vi "CO TCP Packet_v2.0.vi"(7 "TCP Packet Content":string, 13 "Data Array":string[](array[string])) -> (8 "TCP Binary Packet":string)   [LabVIEW 2014]
panel:
  out "array":string[](array[string])
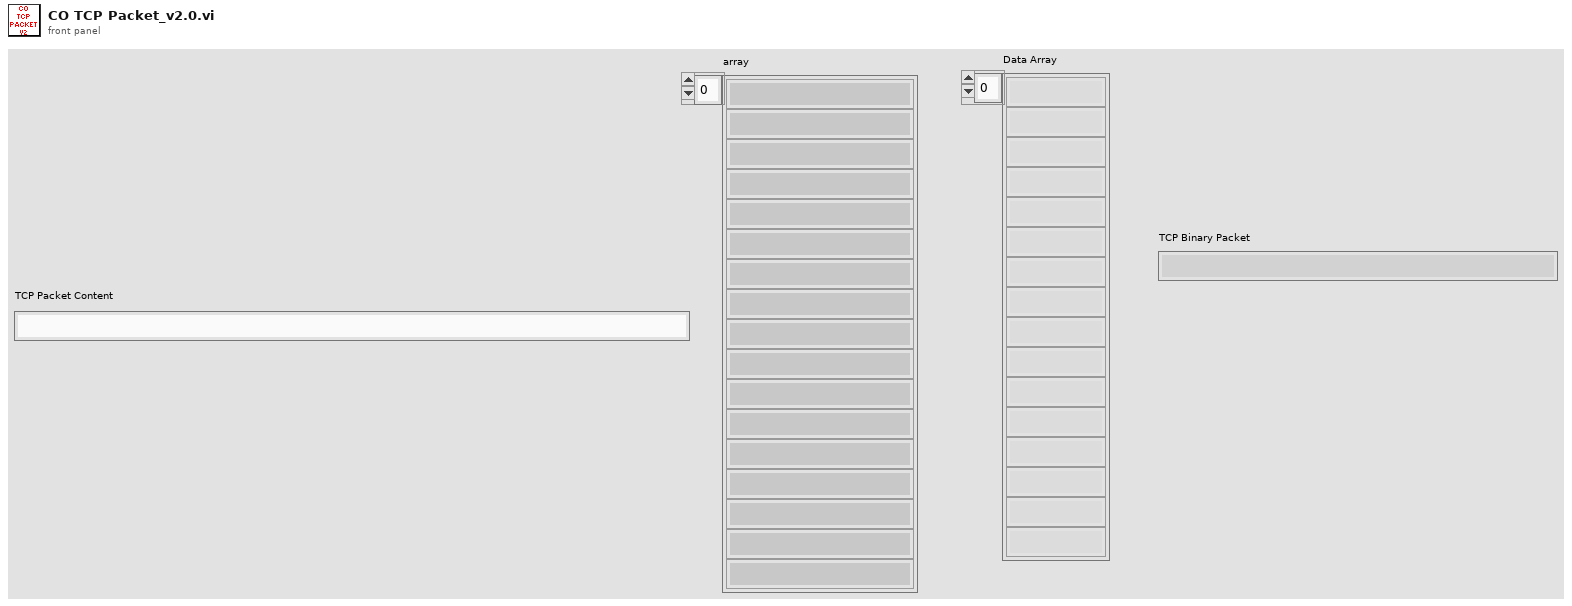
[diagram p1: front panel]
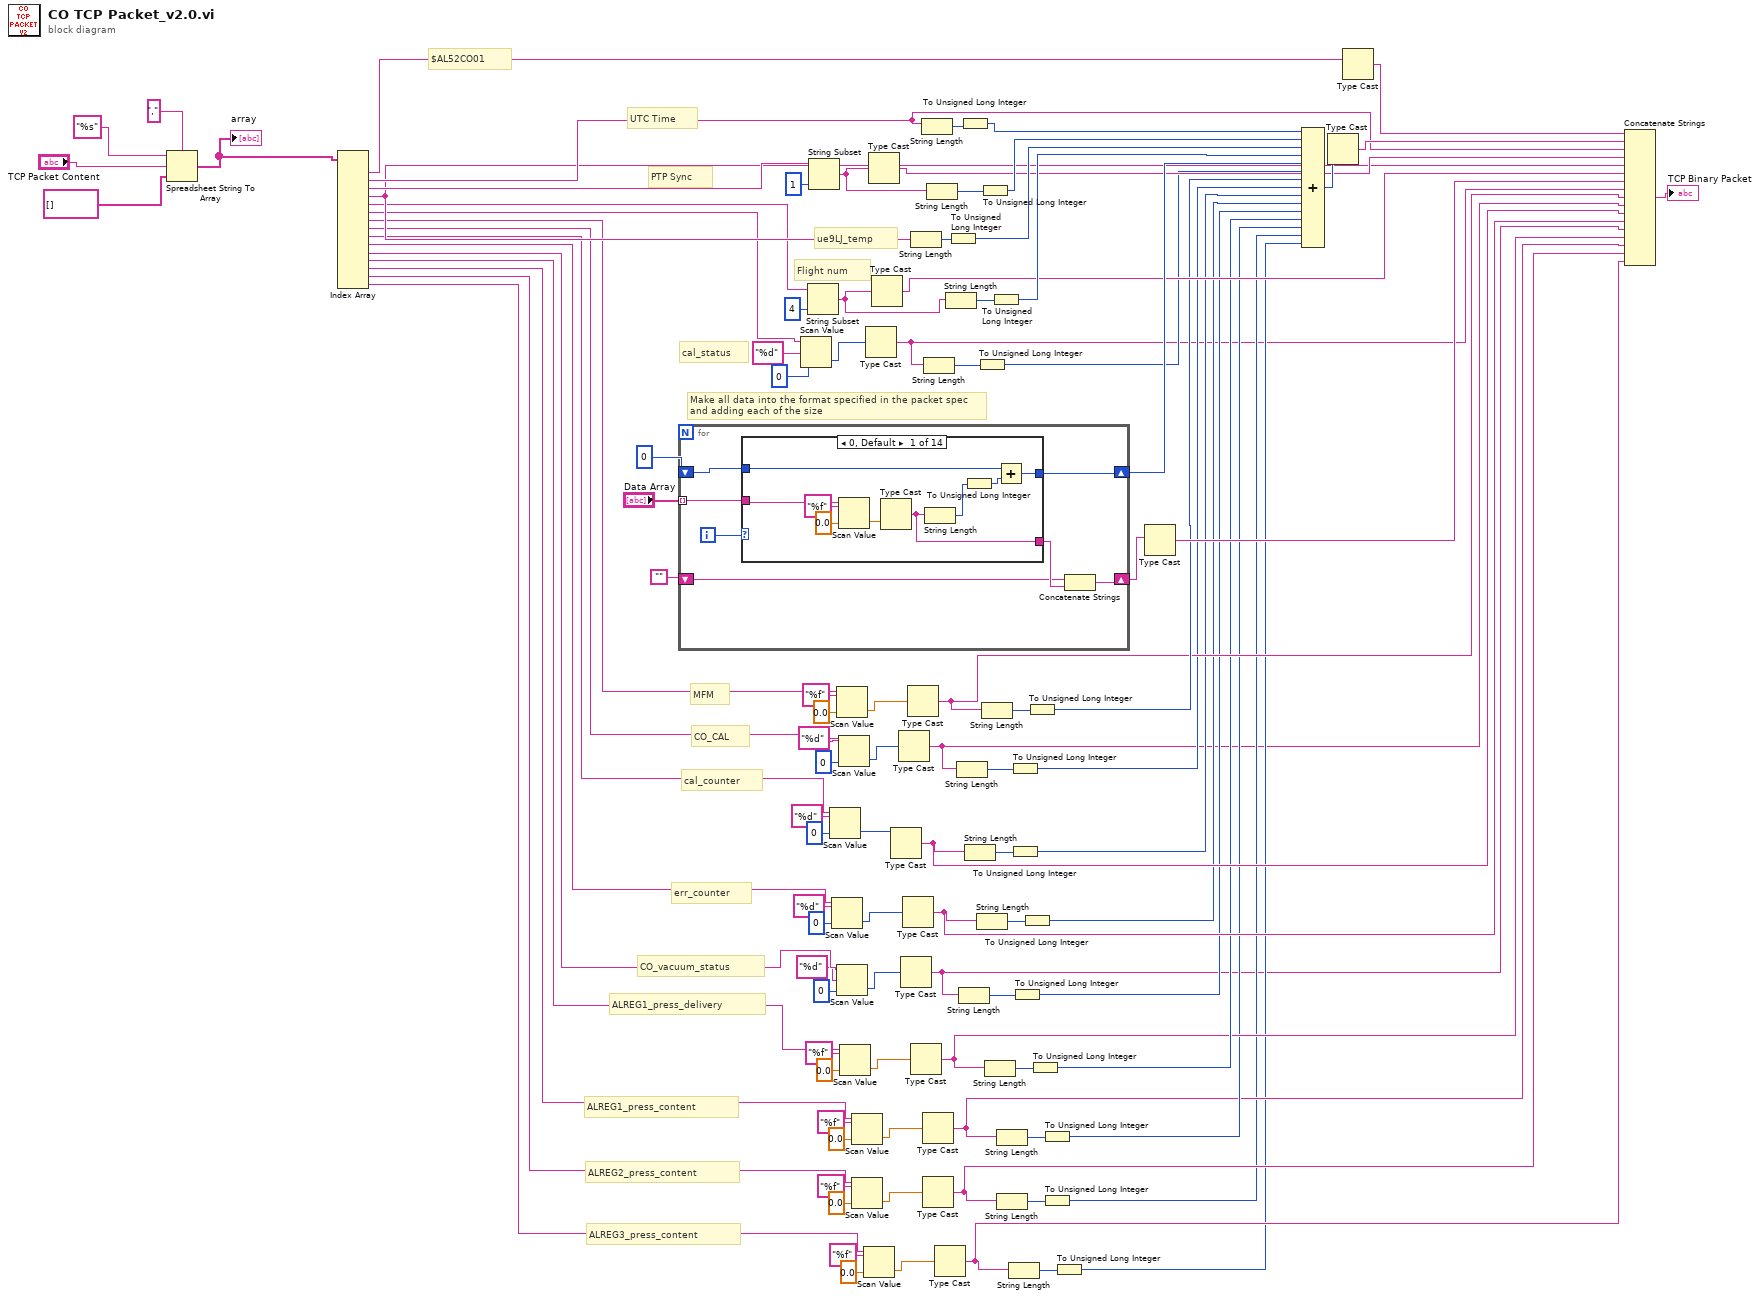
[diagram p0: block diagram]
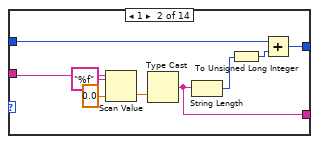
[diagram p2: hidden frame]
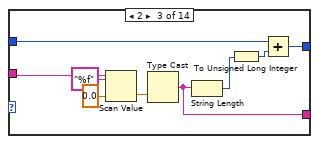
[diagram p3: hidden frame]
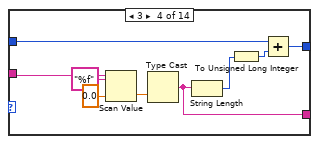
[diagram p4: hidden frame]
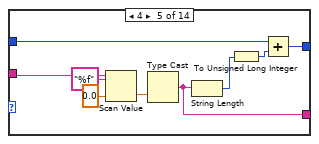
[diagram p5: hidden frame]
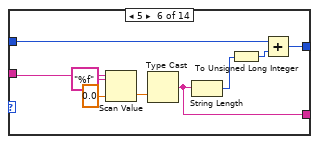
[diagram p6: hidden frame]
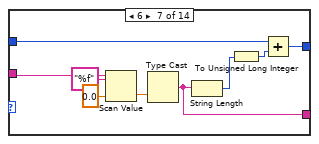
[diagram p7: hidden frame]
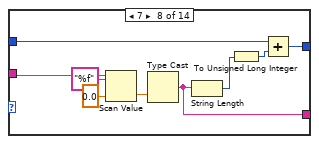
[diagram p8: hidden frame]
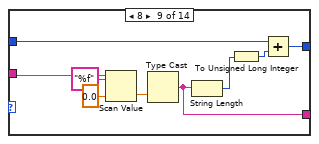
[diagram p9: hidden frame]
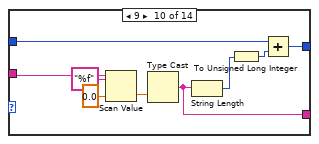
[diagram p10: hidden frame]
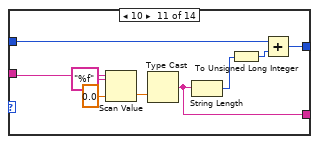
[diagram p11: hidden frame]
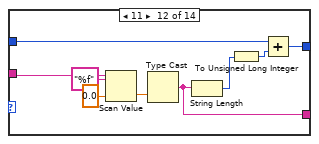
[diagram p12: hidden frame]
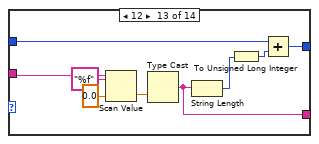
[diagram p13: hidden frame]
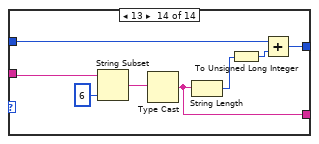
[diagram p14: hidden frame]
diagram:
  # "ALREG3_press_content"
  # "ALREG2_press_content"
  # "ALREG1_press_content"
  # "ALREG1_press_delivery"
  # "CO_vacuum_status"
  # "err_counter"
  # "cal_counter"
  # "CO_CAL"
  # "MFM"
  # "cal_status"
  # "Flight num"
  # "ue9LJ_temp"
  # "PTP Sync"
  # "UTC Time"
  # "$AL52CO01"
  # "Make all data into the format specified in the packet spec\nand adding each of the size"
  n1 = Spreadsheet String To Array(delimiter (Tab)=",", format string="%s", spreadsheet string="TCP Packet Content", array type (2D Dbl)=string[] []) -> (array=w74:string[])
  "array" <- w74
  n2 = Index Array(array=w74) -> (element #1=w73:string, element #2=w72:string, element #3=w71:string, element #4=w70:string, element #5=w69:string, element #6=w10:string, element #7=w64:string, element #8=w15:string, element #9=w34:string, element #10=w31:string, element #11=w4:string, element #12=w27:string, element #13=w24:string, element #14=w20:string, element #15=w18:string)  [unwired: 15 in]
  n3 = for {
    tunnel: "Data Array" -> [w110] mode=indexing
    shift-right: [w108] -> w92
    shift-left: u32 0 -> [w109]
    shift-right: [w107] -> w81
    shift-left: "" -> [w105]
    i -> [w111]
    n4 = case shown="0, Default" w111 {
      tunnel: w110 -> [w118 w127 w136 w145 w154 w163 w172 w181 w190 w199 w208 w217 w226 w230]
      tunnel: w109 -> [w116 w125 w134 w143 w152 w161 w170 w179 w188 w197 w206 w215 w224 w236]
      tunnel: [w113 w122 w131 w140 w149 w158 w167 w176 w185 w194 w203 w212 w221 w233] -> w108
      tunnel: [w112 w121 w130 w139 w148 w157 w166 w175 w184 w193 w202 w211 w220 w232] -> w106
      frame 0, Default {
        n5 = Scan Value(string=w118, format string="%f", default (0 dbl)=sgl 0.0 ("default (0 I32)")) -> (value=w120:sgl)  [unwired: 1 out]
        n6 = Type Cast(x=w120) -> (*(type *) &x=w112:string)  [unwired: 1 in]
        n7 = String Length(string=w112) -> (length=w115:i32)
        n8 = To Unsigned Long Integer(number=w115) -> (unsigned 32bit integer=w114:u32)
        n9 = Add(x=w116, y=w114) -> (x+y=w113:u32)
      }
      frame 1 {
        n10 = Scan Value(string=w127, format string="%f", default (0 dbl)=sgl 0.0 ("default (0 I32)")) -> (value=w129:sgl)  [unwired: 1 out]
        n11 = Type Cast(x=w129) -> (*(type *) &x=w121:string)  [unwired: 1 in]
        n12 = String Length(string=w121) -> (length=w124:i32)
        n13 = To Unsigned Long Integer(number=w124) -> (unsigned 32bit integer=w123:u32)
        n14 = Add(x=w125, y=w123) -> (x+y=w122:u32)
      }
      frame 2 {
        n15 = Scan Value(string=w136, format string="%f", default (0 dbl)=sgl 0.0 ("default (0 I32)")) -> (value=w138:sgl)  [unwired: 1 out]
        n16 = Type Cast(x=w138) -> (*(type *) &x=w130:string)  [unwired: 1 in]
        n17 = String Length(string=w130) -> (length=w133:i32)
        n18 = To Unsigned Long Integer(number=w133) -> (unsigned 32bit integer=w132:u32)
        n19 = Add(x=w134, y=w132) -> (x+y=w131:u32)
      }
      frame 3 {
        n20 = Scan Value(string=w145, format string="%f", default (0 dbl)=sgl 0.0 ("default (0 I32)")) -> (value=w147:sgl)  [unwired: 1 out]
        n21 = Type Cast(x=w147) -> (*(type *) &x=w139:string)  [unwired: 1 in]
        n22 = String Length(string=w139) -> (length=w142:i32)
        n23 = To Unsigned Long Integer(number=w142) -> (unsigned 32bit integer=w141:u32)
        n24 = Add(x=w143, y=w141) -> (x+y=w140:u32)
      }
      frame 4 {
        n25 = Scan Value(string=w154, format string="%f", default (0 dbl)=sgl 0.0 ("default (0 I32)")) -> (value=w156:sgl)  [unwired: 1 out]
        n26 = Type Cast(x=w156) -> (*(type *) &x=w148:string)  [unwired: 1 in]
        n27 = String Length(string=w148) -> (length=w151:i32)
        n28 = To Unsigned Long Integer(number=w151) -> (unsigned 32bit integer=w150:u32)
        n29 = Add(x=w152, y=w150) -> (x+y=w149:u32)
      }
      frame 5 {
        n30 = Scan Value(string=w163, format string="%f", default (0 dbl)=sgl 0.0 ("default (0 I32)")) -> (value=w165:sgl)  [unwired: 1 out]
        n31 = Type Cast(x=w165) -> (*(type *) &x=w157:string)  [unwired: 1 in]
        n32 = String Length(string=w157) -> (length=w160:i32)
        n33 = To Unsigned Long Integer(number=w160) -> (unsigned 32bit integer=w159:u32)
        n34 = Add(x=w161, y=w159) -> (x+y=w158:u32)
      }
      frame 6 {
        n35 = Scan Value(string=w172, format string="%f", default (0 dbl)=sgl 0.0 ("default (0 I32)")) -> (value=w174:sgl)  [unwired: 1 out]
        n36 = Type Cast(x=w174) -> (*(type *) &x=w166:string)  [unwired: 1 in]
        n37 = String Length(string=w166) -> (length=w169:i32)
        n38 = To Unsigned Long Integer(number=w169) -> (unsigned 32bit integer=w168:u32)
        n39 = Add(x=w170, y=w168) -> (x+y=w167:u32)
      }
      frame 7 {
        n40 = Scan Value(string=w181, format string="%f", default (0 dbl)=sgl 0.0 ("default (0 I32)")) -> (value=w183:sgl)  [unwired: 1 out]
        n41 = Type Cast(x=w183) -> (*(type *) &x=w175:string)  [unwired: 1 in]
        n42 = String Length(string=w175) -> (length=w178:i32)
        n43 = To Unsigned Long Integer(number=w178) -> (unsigned 32bit integer=w177:u32)
        n44 = Add(x=w179, y=w177) -> (x+y=w176:u32)
      }
      frame 8 {
        n45 = Scan Value(string=w190, format string="%f", default (0 dbl)=sgl 0.0 ("default (0 I32)")) -> (value=w192:sgl)  [unwired: 1 out]
        n46 = Type Cast(x=w192) -> (*(type *) &x=w184:string)  [unwired: 1 in]
        n47 = String Length(string=w184) -> (length=w187:i32)
        n48 = To Unsigned Long Integer(number=w187) -> (unsigned 32bit integer=w186:u32)
        n49 = Add(x=w188, y=w186) -> (x+y=w185:u32)
      }
      frame 9 {
        n50 = Scan Value(string=w199, format string="%f", default (0 dbl)=sgl 0.0 ("default (0 I32)")) -> (value=w201:sgl)  [unwired: 1 out]
        n51 = Type Cast(x=w201) -> (*(type *) &x=w193:string)  [unwired: 1 in]
        n52 = String Length(string=w193) -> (length=w196:i32)
        n53 = To Unsigned Long Integer(number=w196) -> (unsigned 32bit integer=w195:u32)
        n54 = Add(x=w197, y=w195) -> (x+y=w194:u32)
      }
      frame 10 {
        n55 = Scan Value(string=w208, format string="%f", default (0 dbl)=sgl 0.0 ("default (0 I32)")) -> (value=w210:sgl)  [unwired: 1 out]
        n56 = Type Cast(x=w210) -> (*(type *) &x=w202:string)  [unwired: 1 in]
        n57 = String Length(string=w202) -> (length=w205:i32)
        n58 = To Unsigned Long Integer(number=w205) -> (unsigned 32bit integer=w204:u32)
        n59 = Add(x=w206, y=w204) -> (x+y=w203:u32)
      }
      frame 11 {
        n60 = Scan Value(string=w217, format string="%f", default (0 dbl)=sgl 0.0 ("default (0 I32)")) -> (value=w219:sgl)  [unwired: 1 out]
        n61 = Type Cast(x=w219) -> (*(type *) &x=w211:string)  [unwired: 1 in]
        n62 = String Length(string=w211) -> (length=w214:i32)
        n63 = To Unsigned Long Integer(number=w214) -> (unsigned 32bit integer=w213:u32)
        n64 = Add(x=w215, y=w213) -> (x+y=w212:u32)
      }
      frame 12 {
        n65 = Scan Value(string=w226, format string="%f", default (0 dbl)=sgl 0.0 ("default (0 I32)")) -> (value=w228:sgl)  [unwired: 1 out]
        n66 = Type Cast(x=w228) -> (*(type *) &x=w220:string)  [unwired: 1 in]
        n67 = String Length(string=w220) -> (length=w223:i32)
        n68 = To Unsigned Long Integer(number=w223) -> (unsigned 32bit integer=w222:u32)
        n69 = Add(x=w224, y=w222) -> (x+y=w221:u32)
      }
      frame 13 {
        n70 = String Subset(string=w230, length (rest)=6 ("length (rest)")) -> (substring=w229:string)  [unwired: 1 in]
        n71 = Type Cast(x=w229) -> (*(type *) &x=w232:string)  [unwired: 1 in]
        n72 = String Length(string=w232) -> (length=w235:i32)
        n73 = To Unsigned Long Integer(number=w235) -> (unsigned 32bit integer=w234:u32)
        n74 = Add(x=w236, y=w234) -> (x+y=w233:u32)
      }
    }
    n75 = Concatenate Strings(w105, w106) -> (w107:string)
  }
  n76 = Scan Value(string=w10, format string="%d", default (0 dbl)=u16 0) -> (value=w7:u16)  [unwired: 1 out]
  n77 = String Subset(string=w69, length (rest)=4 ("length (rest)")) -> (substring=w85:string)  [unwired: 1 in]
  n78 = String Subset(string=w71, length (rest)=1 ("length (rest)")) -> (substring=w88:string)  [unwired: 1 in]
  n79 = Scan Value(string=w34, format string="%d", default (0 dbl)=u32 0 ("default (0 I32)")) -> (value=w56:u32)  [unwired: 1 out]
  n80 = Scan Value(string=w31, format string="%d", default (0 dbl)=u32 0 ("default (0 I32)")) -> (value=w52:u32)  [unwired: 1 out]
  n81 = Scan Value(string=w64, format string="%f", default (0 dbl)=sgl 0.0 ("default (0 I32)")) -> (value=w63:sgl)  [unwired: 1 out]
  n82 = Scan Value(string=w4, format string="%d", default (0 dbl)=u16 0 ("length (rest)")) -> (value=w3:u16)  [unwired: 1 out]
  n83 = Scan Value(string=w15, format string="%d", default (0 dbl)=u16 0 ("length (rest)")) -> (value=w11:u16)  [unwired: 1 out]
  n84 = Scan Value(string=w27, format string="%f", default (0 dbl)=sgl 0.0 ("default (0 I32)")) -> (value=w47:sgl)  [unwired: 1 out]
  n85 = Scan Value(string=w24, format string="%f", default (0 dbl)=sgl 0.0 ("default (0 I32)")) -> (value=w43:sgl)  [unwired: 1 out]
  n86 = Scan Value(string=w20, format string="%f", default (0 dbl)=sgl 0.0 ("default (0 I32)")) -> (value=w39:sgl)  [unwired: 1 out]
  n87 = Scan Value(string=w18, format string="%f", default (0 dbl)=sgl 0.0 ("default (0 I32)")) -> (value=w35:sgl)  [unwired: 1 out]
  n88 = Type Cast(x=w7) -> (*(type *) &x=w6:string)  [unwired: 1 in]
  n89 = Type Cast(x=w88) -> (*(type *) &x=w87:string)  [unwired: 1 in]
  n90 = Type Cast(x=w85) -> (*(type *) &x=w86:string)  [unwired: 1 in]
  n91 = Type Cast(x=w56) -> (*(type *) &x=w32:string)  [unwired: 1 in]
  n92 = Type Cast(x=w11) -> (*(type *) &x=w12:string)  [unwired: 1 in]
  n93 = Type Cast(x=w3) -> (*(type *) &x=w2:string)  [unwired: 1 in]
  n94 = Type Cast(x=w52) -> (*(type *) &x=w29:string)  [unwired: 1 in]
  n95 = Type Cast(x=w63) -> (*(type *) &x=w62:string)  [unwired: 1 in]
  n96 = String Length(string=w70) -> (length=w99:i32)
  n97 = Type Cast(x=w47) -> (*(type *) &x=w25:string)  [unwired: 1 in]
  n98 = String Length(string=w72) -> (length=w104:i32)
  n99 = Type Cast(x=w43) -> (*(type *) &x=w22:string)  [unwired: 1 in]
  n100 = Type Cast(x=w39) -> (*(type *) &x=w21:string)  [unwired: 1 in]
  n101 = String Length(string=w6) -> (length=w80:i32)
  n102 = String Length(string=w88) -> (length=w101:i32)
  n103 = Type Cast(x=w35) -> (*(type *) &x=w17:string)  [unwired: 1 in]
  n104 = String Length(string=w85) -> (length=w96:i32)
  n105 = To Unsigned Long Integer(number=w99) -> (unsigned 32bit integer=w98:u32)
  n106 = String Length(string=w12) -> (length=w61:i32)
  n107 = String Length(string=w2) -> (length=w51:i32)
  n108 = To Unsigned Long Integer(number=w104) -> (unsigned 32bit integer=w103:u32)
  n109 = String Length(string=w32) -> (length=w59:i32)
  n110 = To Unsigned Long Integer(number=w80) -> (unsigned 32bit integer=w79:u32)
  n111 = String Length(string=w29) -> (length=w55:i32)
  n112 = To Unsigned Long Integer(number=w101) -> (unsigned 32bit integer=w100:u32)
  n113 = String Length(string=w62) -> (length=w68:i32)
  n114 = String Length(string=w25) -> (length=w50:i32)
  n115 = To Unsigned Long Integer(number=w96) -> (unsigned 32bit integer=w95:u32)
  n116 = String Length(string=w22) -> (length=w46:i32)
  n117 = String Length(string=w21) -> (length=w42:i32)
  n118 = String Length(string=w17) -> (length=w38:i32)
  n119 = To Unsigned Long Integer(number=w61) -> (unsigned 32bit integer=w60:u32)
  n120 = To Unsigned Long Integer(number=w59) -> (unsigned 32bit integer=w33:u32)
  n121 = To Unsigned Long Integer(number=w51) -> (unsigned 32bit integer=w28:u32)
  n122 = To Unsigned Long Integer(number=w55) -> (unsigned 32bit integer=w30:u32)
  n123 = To Unsigned Long Integer(number=w68) -> (unsigned 32bit integer=w67:u32)
  n124 = To Unsigned Long Integer(number=w50) -> (unsigned 32bit integer=w26:u32)
  n125 = To Unsigned Long Integer(number=w46) -> (unsigned 32bit integer=w23:u32)
  n126 = To Unsigned Long Integer(number=w42) -> (unsigned 32bit integer=w19:u32)
  n127 = To Unsigned Long Integer(number=w38) -> (unsigned 32bit integer=w16:u32)
  n128 = Type Cast(x=w81) -> (*(type *) &x=w84:string)  [unwired: 1 in]
  n129 = Compound Arithmetic op=ADD(w103, w100, w98, w95, w92, w79, w67, w60, w33, w30, w28, w26, w23, w19, w16) -> (w90:u32)
  n130 = Type Cast(x=w90) -> (*(type *) &x=w89:string)  [unwired: 1 in]
  n131 = Type Cast(x=w73) -> (*(type *) &x=w91:string)  [unwired: 1 in]
  n132 = Concatenate Strings(w91, w89, w72, w87, w70, w86, w84, w6, w62, w12, w32, w29, w2, w25, w22, w21, w17) -> (→"TCP Binary Packet":string)
